vi "warefrom de escritura.vi"() -> ()   [LabVIEW 2020]
panel:
  in  "stop":bool
  out "grafico de señal":dynamicdata(graph)
  out "alarma":bool
  in  "lim":dbl(slide) scale=0.0..100.0
  in  "temp":dbl
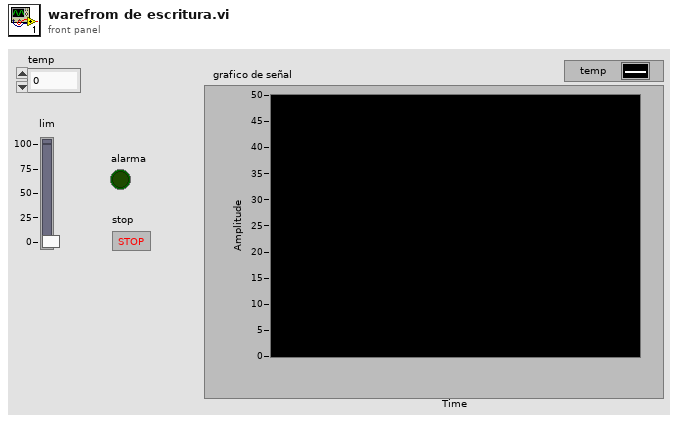
[diagram p1: front panel]
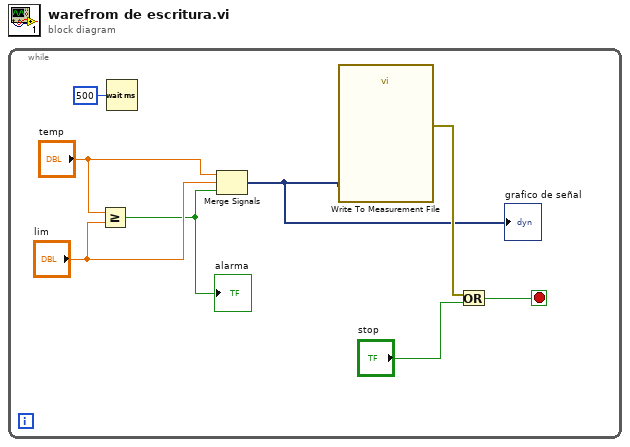
[diagram p0: block diagram]
diagram:
  n1 = while {
    stop <- w5 stop-if-true
    n2 = Greater Or Equal?(x="temp", y="lim") -> (x >= y?=w1:bool)
    "alarma" <- w1
    n3 = Wait (ms)(milliseconds to wait=u32 500) -> ()  [unwired: 1 out]
    n4 = Merge Signals("temp", "lim", w1) -> (w4:dynamicdata)
    "grafico de señal" <- w4
    n5 = call "Write To Measurement File"("Signals"=w4) -> ("error out"=w6:errorcluster)  [unwired: 16 in, 2 out]
    n6 = Or(x=w6, y="stop") -> (x .or. y?=w5:bool)
  }
